vi "Add Item.vi"(7 "Action":T3, 8 "error in (no error)":errorcluster, 11 "SE UI cluster in":T1={"Node Ptr"=18446744073709551615, "Add"=refnum, "Remove"=refnum, "Registers ListBox"=refnum} {"Node Ptr" format="%.0x"}) -> (0 "error out":errorcluster, 3 "SE UI cluster out":T1={"Node Ptr"=18446744073709551615, "Add"=refnum, "Remove"=refnum, "Registers ListBox"=refnum} {"Node Ptr" format="%.0x"})   [LabVIEW 2019, in "FPGA Addon System Explorer.lvlib"]
uses:
  FPGA Addon System Explorer.lvlib
  Types/Channel Type.ctl
  Types/SE UI Cluster.ctl
  <vilib>/NI VeriStand/Custom Device API/Custom Device Item Ref.ctl
  <vilib>/NI VeriStand/Custom Device API/Custom Device API.lvlib
  APIs/Scripting API/Scripting API.lvlib
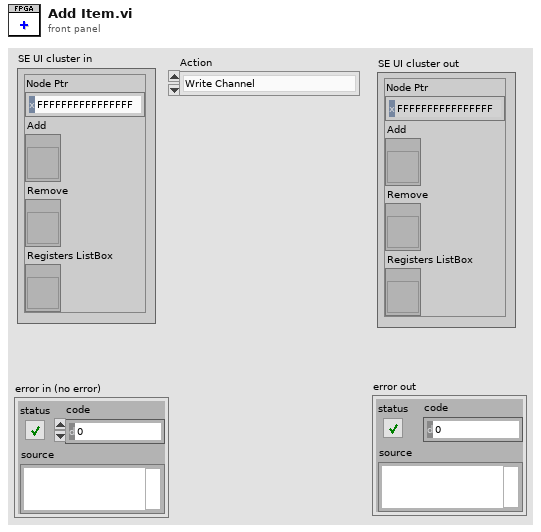
[diagram p1: front panel]
types:
  T1 = typedef "FPGA Addon System Explorer.lvlib/SE UI Cluster.ctl" = cluster{"Node Ptr":T2, "Add":refnum<vi>, "Remove":refnum<vi>, "Registers ListBox":refnum<vi>}
  T2 = typedef "Custom Device API.lvlib/Custom Device Item Ref.ctl" = u64
  T3 = typedef "FPGA Addon System Explorer.lvlib/Channel Type.ctl" = enum16{"Write Channel", "Read Channel", "Write Waveform", "Read Waveform"}
  T4 = enum32{"invalid app kind", "Development System", "Run Time System", "Student Edition", "Embedded LabVIEW", "Evaluation", "Custom"}
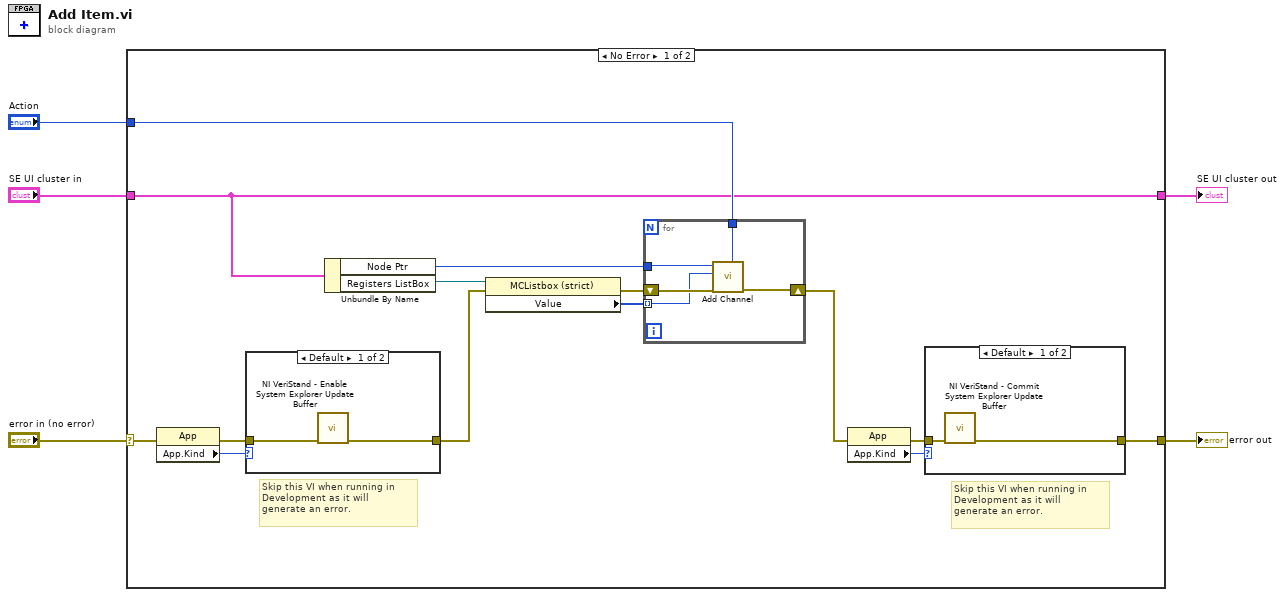
[diagram p0: block diagram]
diagram:
  n1 = case shown="No Error" "error in (no error)" {
    selector: "error in (no error)" -> [w9 w32]
    tunnel: "SE UI cluster in" -> [w7 w31]
    tunnel: "Action" -> [w8 _]
    tunnel: [w6 w32] -> w3
    tunnel: [w7 w31] -> w1
    frame No Error {
      # "Skip this VI when running in Development as it will generate an error."
      # "Skip this VI when running in Development as it will generate an error."
      n2 = property class="App"(error in=w9) -> (error out=w17:errorcluster, "App.Kind"=w16:T4)  [unwired: 1 in, 1 out]
      n3 = case shown="Default" w16 {
        tunnel: [w26 w27] -> w13
        tunnel: w17 -> [w25 w27]
        frame Default {
          n4 = call <vilib>:"NI VeriStand - Enable System Explorer Update Buffer.vi"("error in (no error)"=w25) -> ("error out"=w26:errorcluster)  [unwired: 10 in]
        }
        frame "Development System" {
        }
      }
      n5 = Unbundle By Name(w7) -> ("Node Ptr"=w15:T2, "Registers ListBox"=w14:refnum<vi>)
      n6 = property class="MCListbox (strict)"(reference=w14, error in=w13) -> (error out=w12:errorcluster, "Value"=w11:i32[])  [unwired: 1 out]
      n7 = for {
        tunnel: w11 -> [w20] mode=indexing
        tunnel: w15 -> [w24]
        shift-right: [w22] -> w10
        shift-left: w12 -> [w23]
        tunnel: w8 -> [w21]
        n8 = call "Add Channel.vi"("Action"=w21, "error in (no error)"=w23, "Register Index"=w20, "Node Ptr in"=w24) -> ("error out"=w22:errorcluster)  [unwired: 6 in, 1 out]
      }
      n9 = property class="App"(error in=w10) -> (error out=w19:errorcluster, "App.Kind"=w18:T4)  [unwired: 1 in, 1 out]
      n10 = case shown="Default" w18 {
        tunnel: [w29 w30] -> w6
        tunnel: w19 -> [w28 w30]
        frame Default {
          n11 = call <vilib>:"NI VeriStand - Commit System Explorer Update Buffer.vi"("error in (no error)"=w28) -> ("error out"=w29:errorcluster)  [unwired: 10 in]
        }
        frame "Development System" {
        }
      }
    }
    frame Error {
    }
  }
  "error out" <- w3
  "SE UI cluster out" <- w1
